vi "_Translator.vi"(0 "Input":variant, 11 "error in (no error)":errorcluster) -> (4 "Output":variant, 15 "error out":errorcluster)   [LabVIEW 2014, in "Arduino SoftwareSerial Wrapper.lvlib"]
doc: "An example of how to create the Translator to convert the LabVIEW VIs to Arduino C code."
uses:
  <vilib>/Aledyne-TSXperts/Arduino Compatible Compiler for LabVIEW/addons/Arduino SoftwareSerial Wrapper/Arduino SoftwareSerial Wrapper.lvlib
panel:
  out "Outputs":string[](array[string])
  out "Inputs":string[](array[string])
  out "Output Datatypes":string[](array[string])
  out "Input Datatypes":string[](array[string])
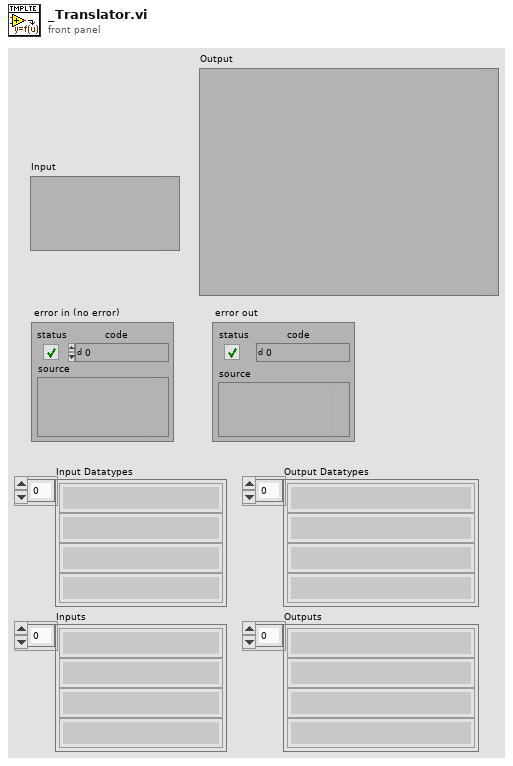
[diagram p1: front panel]
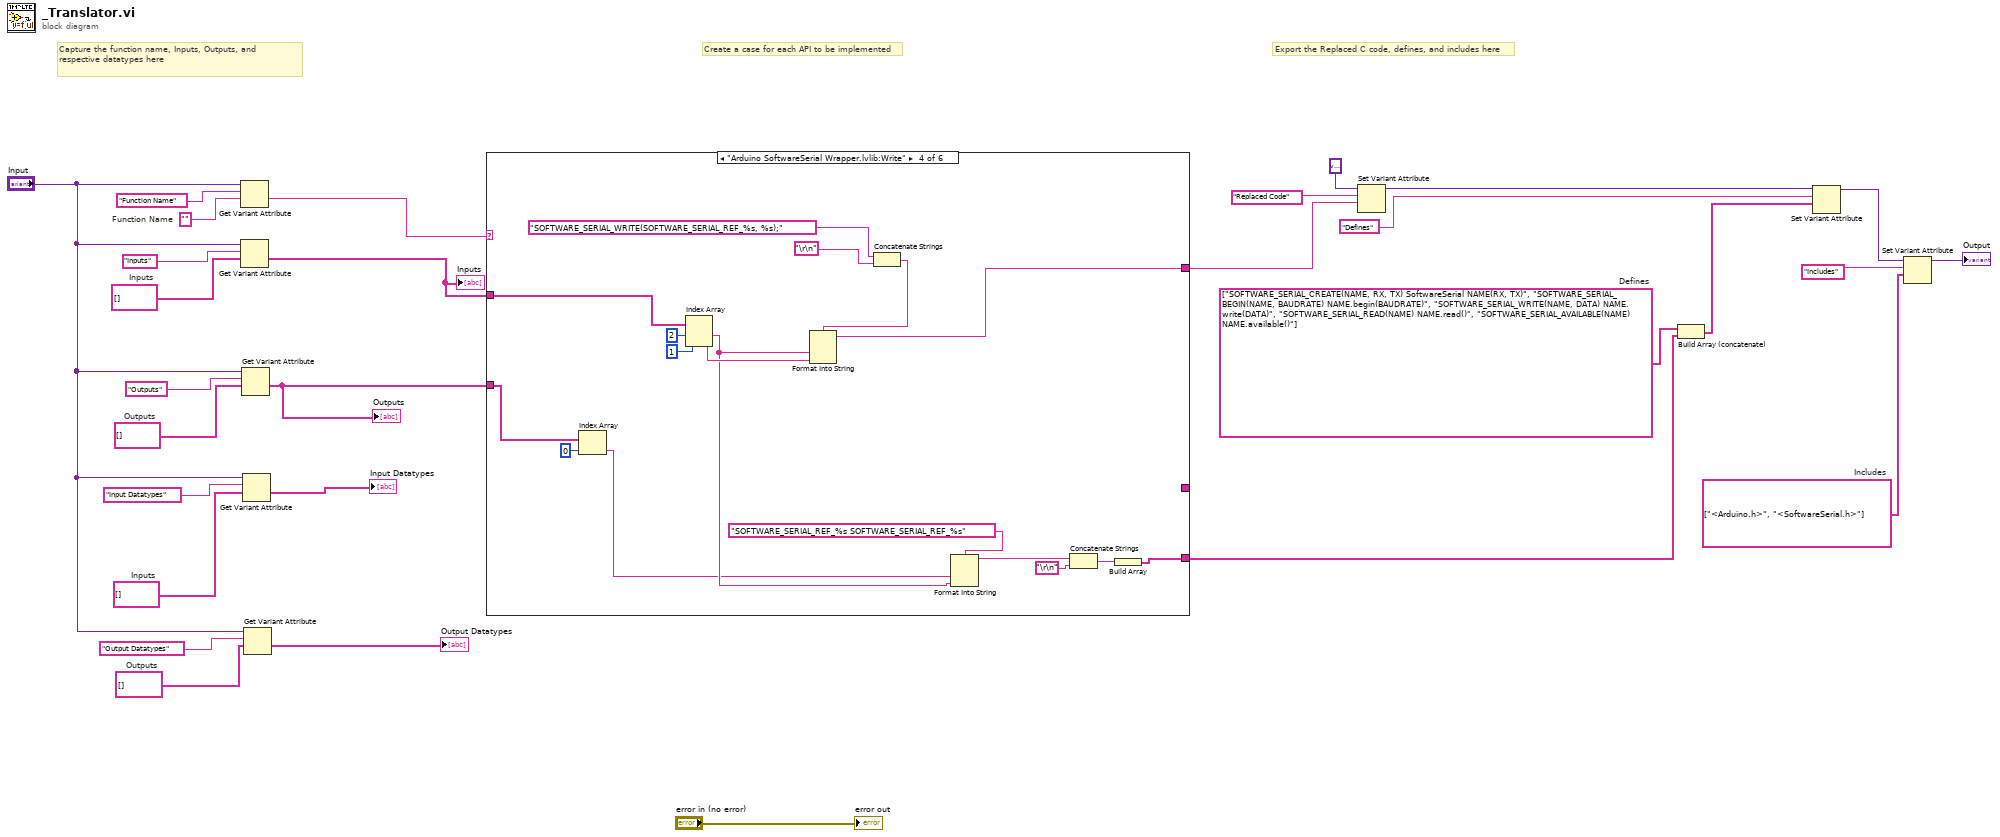
[diagram p0: block diagram]
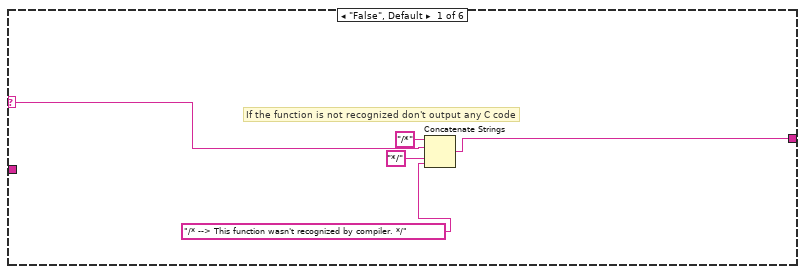
[diagram p2: hidden frame]
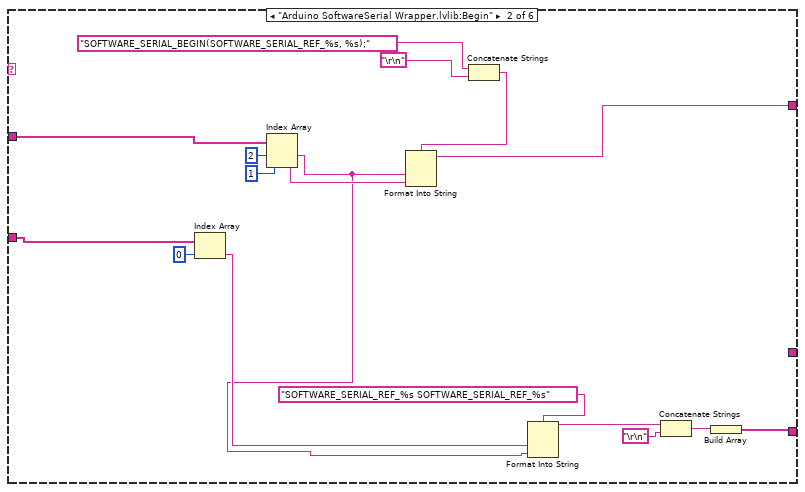
[diagram p3: hidden frame]
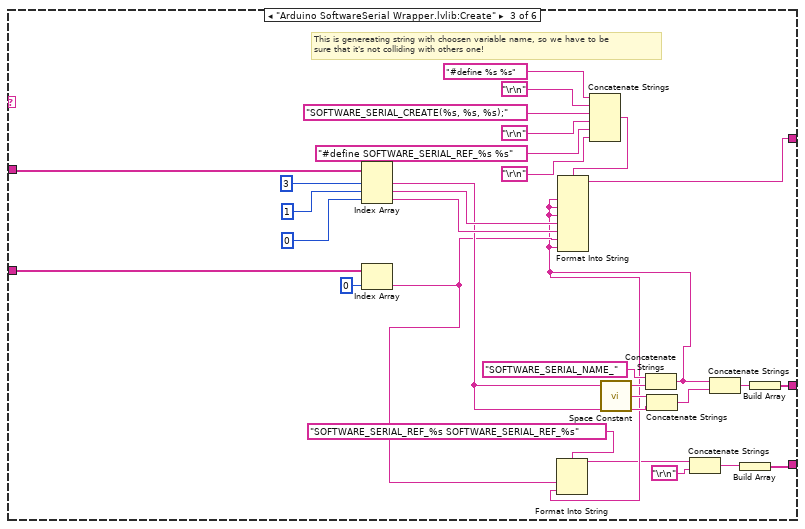
[diagram p4: hidden frame]
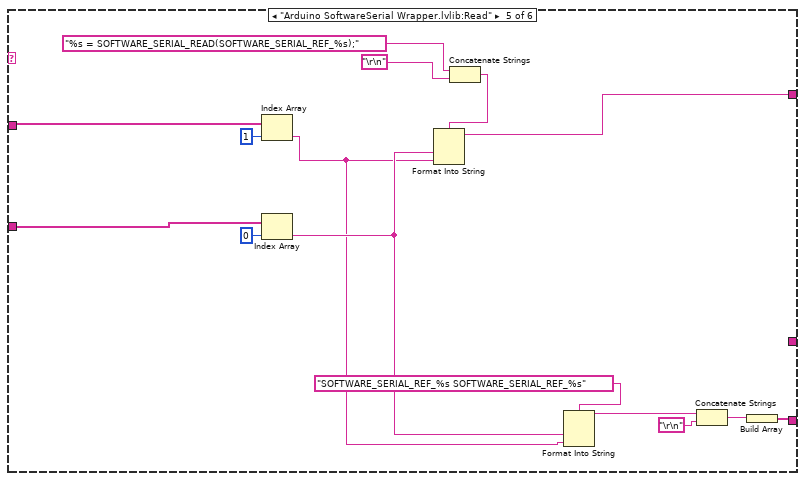
[diagram p5: hidden frame]
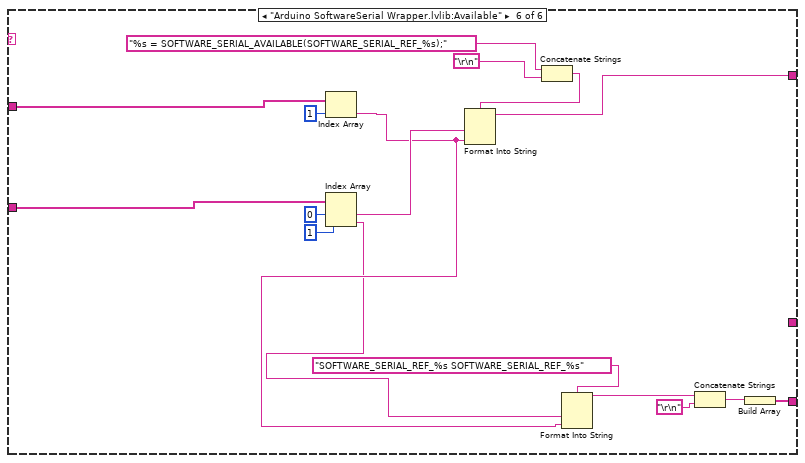
[diagram p6: hidden frame]
diagram:
  w3 = string[] ["SOFTWARE_SERIAL_CREATE(NAME, RX, TX) SoftwareSerial NAME(RX, TX)", "SOFTWARE_SERIAL_BEGIN(NAME, BAUDRATE) NAME.begin(BAUDRATE)", "SOFTWARE_SERIAL_WRITE(NAME, DATA) NAME.write(DATA)", "SOFTWARE_SERIAL_READ(NAME) NAME.read()", "SOFTWARE_SERIAL_AVAILABLE(NAME) NAME.available()"]  # Defines
  w15 = string[] []  # Outputs
  w16 = string[] []  # Inputs
  w20 = string[] ["<Arduino.h>", "<SoftwareSerial.h>"]  # Includes
  w25 = string[] []  # Outputs
  w26 = string[] []  # Inputs
  w27 = ""  # Function Name
  # "Capture the function name, Inputs, Outputs, and respective datatypes here"
  # "Export the Replaced C code, defines, and includes here"
  # "Create a case for each API to be implemented"
  n1 = Get Variant Attribute(Variant="Input", name="Function Name", default value (empty Variant)=w27) -> (value=w22:string)  [unwired: 1 in, 3 out]
  n2 = Get Variant Attribute(Variant="Input", name="Inputs", default value (empty Variant)=w26) -> (value=w11:string[])  [unwired: 1 in, 3 out]
  "Inputs" <- w11
  n3 = Get Variant Attribute(Variant="Input", name="Outputs", default value (empty Variant)=w25) -> (value=w12:string[])  [unwired: 1 in, 3 out]
  "Outputs" <- w12
  n4 = Get Variant Attribute(Variant="Input", name="Input Datatypes", default value (empty Variant)=w16) -> (value=→"Input Datatypes":string[])  [unwired: 1 in, 3 out]
  n5 = Get Variant Attribute(Variant="Input", name="Output Datatypes", default value (empty Variant)=w15) -> (value=→"Output Datatypes":string[])  [unwired: 1 in, 3 out]
  n6 = case shown="\"Arduino SoftwareSerial Wrapper.lvlib:Write\"" w22 {
    selector: w22 -> [w32 _ _ _ _ _]
    tunnel: [w30 w50 w77 w95 w110 w127] -> w21
    tunnel: w11 -> [_ w51 w78 w96 w111 w129]
    tunnel: w12 -> [_ w37 w73 w82 w112 w128]
    tunnel: [_ _ w75 _ _ _] -> _
    tunnel: [_ w39 w55 w85 w100 w117] -> w1
    frame "False", Default {
      # "If the function is not recognized don't output any C code"
      n7 = Concatenate Strings("/*" ("name"), w32, "*/" ("name"), "/* --> This function wasn't recognized by compiler. */" ("name")) -> (w30:string)
    }
    frame "Arduino SoftwareSerial Wrapper.lvlib:Begin" {
      n8 = Index Array(array=w37, index=0) -> (element=w36:string)
      n9 = Index Array(array=w51, index #1=2 ("index"), index #2=1 ("index")) -> (element #1=w35:string, element #2=w49:string)
      n10 = Concatenate Strings("SOFTWARE_SERIAL_BEGIN(SOFTWARE_SERIAL_REF_%s, %s);" ("name"), "\r\n") -> (w44:string)
      n11 = Format Into String(format string=w44, w35, w49) -> (resulting string=w50:string)  [unwired: 2 in, 1 out]
      n12 = Format Into String(format string="SOFTWARE_SERIAL_REF_%s SOFTWARE_SERIAL_REF_%s" ("name"), w36, w35) -> (resulting string=w42:string)  [unwired: 2 in, 1 out]
      n13 = Concatenate Strings(w42, "\r\n") -> (w41:string)
      n14 = Build Array(w41) -> (w39:string[])
    }
    frame "Arduino SoftwareSerial Wrapper.lvlib:Create" {
      # "This is genereating string with choosen variable name, so we have to be\nsure that it's not colliding with others one!"
      n15 = Index Array(array=w78, index #1=3 ("index"), index #2=1 ("index"), index #3=0 ("index")) -> (element #1=w59:string, element #2=w68:string, element #3=w67:string)
      n16 = Index Array(array=w73, index=0) -> (element=w57:string)
      n17 = Concatenate Strings("#define %s %s" ("name"), "\r\n", "SOFTWARE_SERIAL_CREATE(%s, %s, %s);" ("name"), "\r\n", "#define SOFTWARE_SERIAL_REF_%s %s" ("name"), "\r\n") -> (w66:string)
      n18 = call <vilib>:"Space Constant.vi"() -> ("String"=w71:string)
      n19 = Concatenate Strings("SOFTWARE_SERIAL_NAME_" ("element"), w59) -> (w56:string)
      n20 = Format Into String(format string="SOFTWARE_SERIAL_REF_%s SOFTWARE_SERIAL_REF_%s" ("name"), w57, w56) -> (resulting string=w53:string)  [unwired: 2 in, 1 out]
      n21 = Format Into String(format string=w66, w56, w56, w56, w68, w67, w57, w56) -> (resulting string=w77:string)  [unwired: 2 in, 1 out]
      n22 = Concatenate Strings(w71, w59) -> (w69:string)
      n23 = Concatenate Strings(w53, "\r\n") -> (w54:string)
      n24 = Concatenate Strings(w56, w69) -> (w70:string)
      n25 = Build Array(w54) -> (w55:string[])
      n26 = Build Array(w70) -> (w75:string[])
    }
    frame "Arduino SoftwareSerial Wrapper.lvlib:Write" {
      n27 = Index Array(array=w82, index=0) -> (element=w81:string)
      n28 = Index Array(array=w96, index #1=2 ("index"), index #2=1 ("index")) -> (element #1=w84:string, element #2=w97:string)
      n29 = Concatenate Strings("SOFTWARE_SERIAL_WRITE(SOFTWARE_SERIAL_REF_%s, %s);" ("name"), "\r\n") -> (w90:string)
      n30 = Format Into String(format string=w90, w84, w97) -> (resulting string=w95:string)  [unwired: 2 in, 1 out]
      n31 = Format Into String(format string="SOFTWARE_SERIAL_REF_%s SOFTWARE_SERIAL_REF_%s" ("name"), w81, w84) -> (resulting string=w88:string)  [unwired: 2 in, 1 out]
      n32 = Concatenate Strings(w88, "\r\n") -> (w87:string)
      n33 = Build Array(w87) -> (w85:string[])
    }
    frame "Arduino SoftwareSerial Wrapper.lvlib:Read" {
      n34 = Index Array(array=w111, index=1) -> (element=w98:string)
      n35 = Index Array(array=w112, index=0) -> (element=w99:string)
      n36 = Concatenate Strings("%s = SOFTWARE_SERIAL_READ(SOFTWARE_SERIAL_REF_%s);" ("name"), "\r\n") -> (w105:string)
      n37 = Format Into String(format string=w105, w99, w98) -> (resulting string=w110:string)  [unwired: 2 in, 1 out]
      n38 = Format Into String(format string="SOFTWARE_SERIAL_REF_%s SOFTWARE_SERIAL_REF_%s" ("name"), w99, w98) -> (resulting string=w102:string)  [unwired: 2 in, 1 out]
      n39 = Concatenate Strings(w102, "\r\n") -> (w103:string)
      n40 = Build Array(w103) -> (w100:string[])
    }
    frame "Arduino SoftwareSerial Wrapper.lvlib:Available" {
      n41 = Index Array(array=w129, index=1) -> (element=w115:string)
      n42 = Index Array(array=w128, index #1=0 ("index"), index #2=1 ("index")) -> (element #1=w116:string, element #2=w113:string)
      n43 = Concatenate Strings("%s = SOFTWARE_SERIAL_AVAILABLE(SOFTWARE_SERIAL_REF_%s);" ("name"), "\r\n") -> (w123:string)
      n44 = Format Into String(format string=w123, w116, w115) -> (resulting string=w127:string)  [unwired: 2 in, 1 out]
      n45 = Format Into String(format string="SOFTWARE_SERIAL_REF_%s SOFTWARE_SERIAL_REF_%s" ("name"), w113, w115) -> (resulting string=w119:string)  [unwired: 2 in, 1 out]
      n46 = Concatenate Strings(w119, "\r\n") -> (w120:string)
      n47 = Build Array(w120) -> (w117:string[])
    }
  }
  n48 = Set Variant Attribute(Variant=variant ("variant"), name="Replaced Code", value=w21) -> (Variant out=w9:variant)  [unwired: 1 in, 2 out]
  n49 = Build Array (concatenate)(w3, w1) -> (w2:string[])
  n50 = Set Variant Attribute(Variant=w9, name="Defines", value=w2) -> (Variant out=w8:variant)  [unwired: 1 in, 2 out]
  n51 = Set Variant Attribute(Variant=w8, name="Includes", value=w20) -> (Variant out=→"Output":variant)  [unwired: 1 in, 2 out]
  "error out" <- "error in (no error)"
